vi "Read Offline Log.vi"(8 "error in (no error)":errorcluster, 11 "Log.Litho in":refnum<class "Log.Litho.lvclass">) -> (0 "error out":errorcluster, 2 "Offline Log":string, 3 "Log.Litho out":refnum<class "Log.Litho.lvclass">)   [LabVIEW 2019, in "Log.Litho.lvclass"]
uses:
  Log.Litho.lvclass
  Log.Litho.lvclass/Log.Litho.ctl
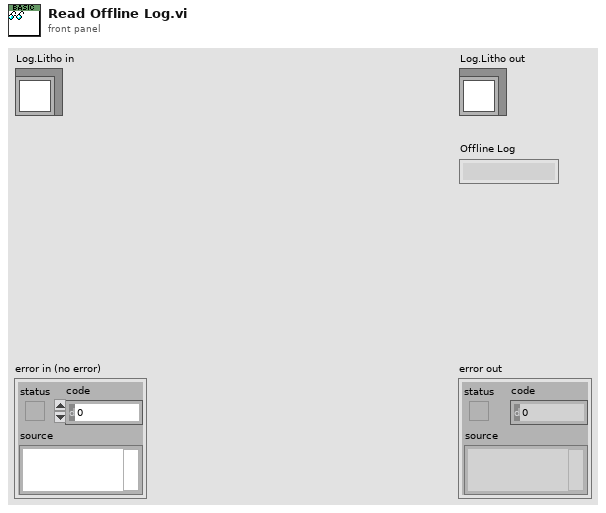
[diagram p1: front panel]
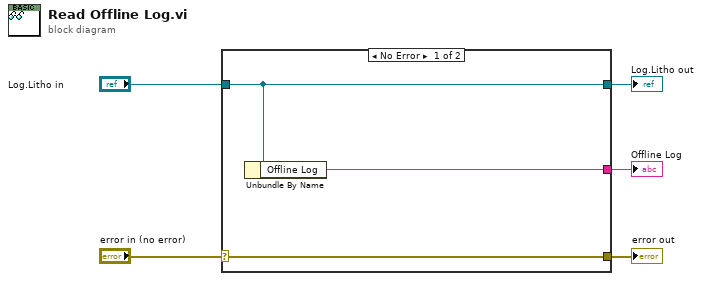
[diagram p0: block diagram]
diagram:
  n1 = case shown="No Error" "error in (no error)" {
    selector: "error in (no error)" -> [w8 w9]
    tunnel: [w8 w9] -> w4
    tunnel: [w7 w10] -> w2
    tunnel: "Log.Litho in" -> [w7 w10]
    tunnel: [w6 _] -> w1
    frame No Error {
      n2 = Unbundle By Name(w7) -> ("Offline Log"=w6:string)
    }
    frame Error {
    }
  }
  "error out" <- w4
  "Log.Litho out" <- w2
  "Offline Log" <- w1
